vi "isLeapYear (Poly).vi"   [LabVIEW 2018]
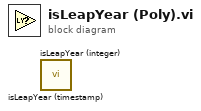
[diagram p0: block diagram]
diagram:
  n1 = call <vilib>:"isLeapYear (timestamp).vi"() -> ()  [unwired: 9 in, 1 out]
  n2 = call <vilib>:"isLeapYear (integer).vi"() -> ()  [unwired: 9 in, 1 out]
